vi "VPA QC Update Flow Rate Volume Pumped.vi"(6 "ReqStp?":bool, 7 "MS Time":u32, 9 "MLtot":refnum<vi>, 10 "Flow Rate Data In":T1(array[cluster]), 11 "Test #":i8) -> (0 "Elapsed Time":dbl, 1 "Volume":dbl, 2 "Flow Data Out":T1(array[cluster]))   [LabVIEW 2013]
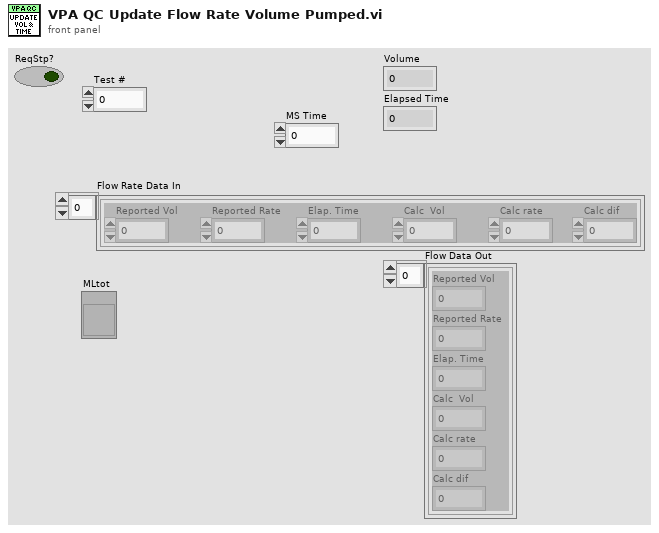
[diagram p1: front panel]
types:
  T1 = cluster{"Reported Vol":dbl, "Reported Rate":dbl, "Elap. Time":dbl, "Calc  Vol":dbl, "Calc rate":dbl, "Calc dif":dbl}[]
  T2 = cluster{"Reported Vol":dbl, "Reported Rate":dbl, "Elap. Time":dbl, "Calc  Vol":dbl, "Calc rate":dbl, "Calc dif":dbl}
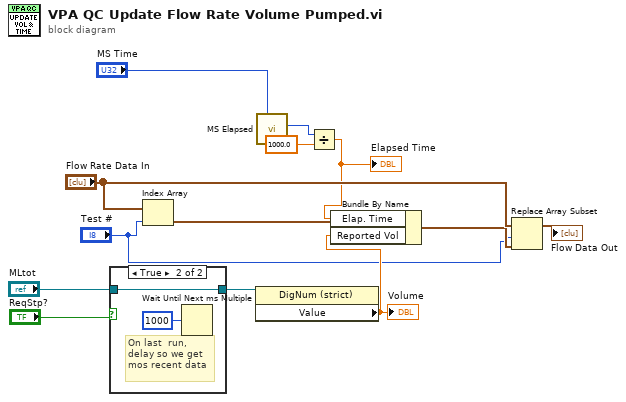
[diagram p0: block diagram]
diagram:
  n1 = case shown="True" "ReqStp?" {
    tunnel: "MLtot" -> [w14 w16]
    tunnel: [w14 w16] -> w12
    frame False {
    }
    frame True {
      # "On last  run, \ndelay so we get \nmos recent data"
      n2 = Wait Until Next ms Multiple(millisecond multiple=u32 1000) -> ()  [unwired: 1 out]
    }
  }
  n3 = Index Array(array="Flow Rate Data In", index="Test #") -> (element=w10:T2)
  n4 = property class="DigNum (strict)"(reference=w12) -> ("Value"=w9:dbl)  [unwired: 1 in, 2 out]
  "Volume" <- w9
  n5 = call "MS Elapsed.vi"("ms in"="MS Time") -> ("elapsed ms"=w3:u32)  [unwired: 9 in, 1 out]
  n6 = Divide(x=w3, y=1000.0) -> (x/y=w1:dbl)
  "Elapsed Time" <- w1
  n7 = Bundle By Name(cluster=w10, "Elap. Time"=w1, "Reported Vol"=w9) -> (w7:T2)
  n8 = Replace Array Subset(array="Flow Rate Data In", new element=w7, index="Test #") -> (→"Flow Data Out":T1)
